vi "GetPoint.vi"(8 "error in (no error)":errorcluster, 11 "Picture in":refnum<class "Image.lvclass">) -> (0 "error out":errorcluster, 2 "Point":refnum<class "Point.lvclass">, 3 "Picture out":refnum<class "Image.lvclass">)   [LabVIEW 2021, in "Picture2D.lvlib" / "Image.lvclass"]
uses:
  Image.lvclass
  Picture2D/Picture2D.lvclass
  Point/Point.lvclass
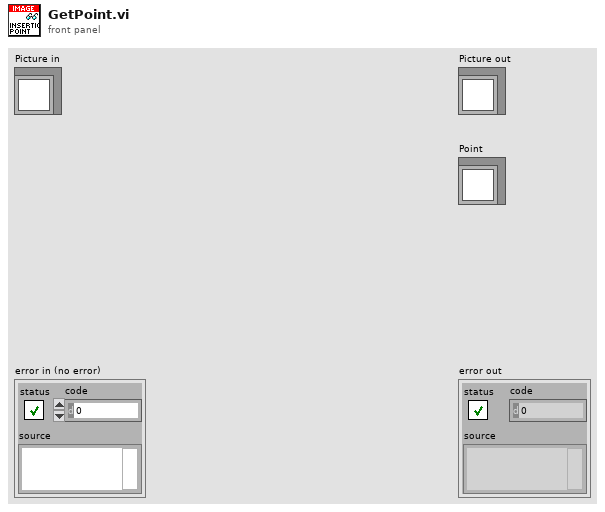
[diagram p1: front panel]
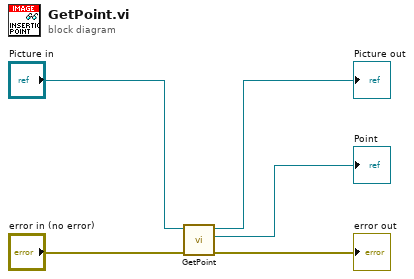
[diagram p0: block diagram]
diagram:
  n1 = call-parent "GetPoint.vi"("error in (no error)"="error in (no error)", "Picture2D in"="Picture in") -> ("error out"=→"error out":errorcluster, "Point"=→"Point":refnum<class "Point.lvclass">, "Picture2D out"=→"Picture out":refnum<class "Image.lvclass">)  [unwired: 7 in]
